vi "deletetitel.vi"(8 "pos":dbl, 9 "symbole":dbl[](array[numeric]), 10 "playlist":string[](array[string]), 11 "pfade":string[](array[string])) -> (1 "symbole out":dbl[](array[numeric]), 2 "playlist out":string[](array[string]), 3 "pfade out":string[](array[string]))   [LabVIEW 2012]
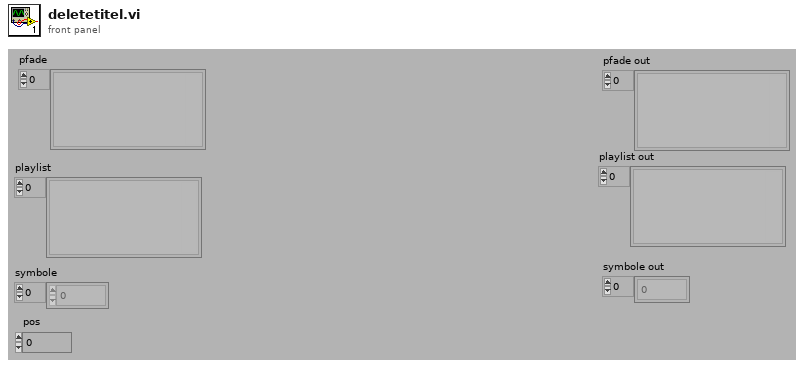
[diagram p1: front panel]
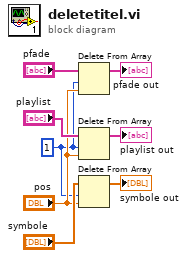
[diagram p0: block diagram]
diagram:
  w2 = 1 ("Länge")
  n1 = Delete From Array(array="pfade", length=w2, index="pos") -> (array with subset deleted=→"pfade out":string[])  [unwired: 1 out]
  n2 = Delete From Array(array="playlist", length=w2, index="pos") -> (array with subset deleted=→"playlist out":string[])  [unwired: 1 out]
  n3 = Delete From Array(array="symbole", length=w2, index="pos") -> (array with subset deleted=→"symbole out":dbl[])  [unwired: 1 out]
